vi "DQMH_API_Get All Events in Module.vi"(7 "include all events (F)":bool, 8 "error in (no error)":errorcluster, 11 "Module Info":T1) -> (0 "error out":errorcluster, 3 "Event Info":T2(array[cluster]))   [LabVIEW 2020]
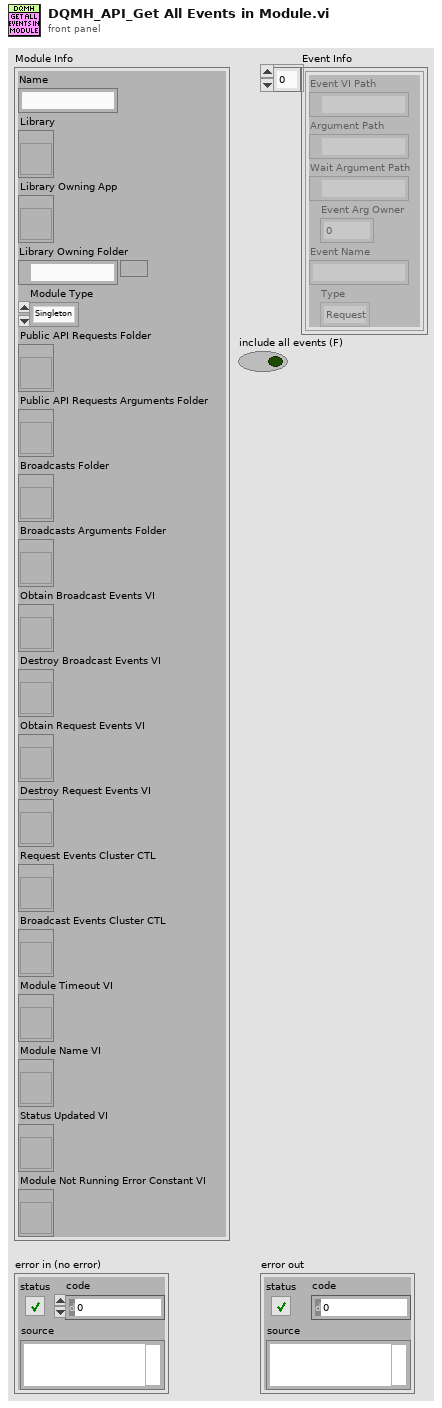
[diagram p1: front panel]
types:
  T1 = cluster{"Name":string, "Library":refnum<vi>, "Library Owning App":refnum<vi>, "Library Owning Folder":path, "Module Type":enum16{"Singleton", "Cloneable"}, "Public API Requests Folder":refnum<vi>, "Public API Requests Arguments Folder":refnum<vi>, "Broadcasts Folder":refnum<vi>, "Broadcasts Arguments Folder":refnum<vi>, "Obtain Broadcast Events VI":refnum<vi>, "Destroy Broadcast Events VI":refnum<vi>, "Obtain Request Events VI":refnum<vi>, "Destroy Request Events VI":refnum<vi>, "Request Events Cluster CTL":refnum<vi>, "Broadcast Events Cluster CTL":refnum<vi>, "Module Timeout VI":refnum<vi>, "Module Name VI":refnum<vi>, "Status Updated VI":refnum<vi>, "Module Not Running Error Constant VI":refnum<vi>}
  T2 = cluster{"Event VI Path":path, "Argument Path":path, "Wait Argument Path":path, "Event Arg Owner":i32, "Event Name":string, "Type":enum16{"Request", "Broadcast", "Both"}}[]
  T3 = typedef "DQMH New Unit Test.lvlib/Event Info.ctl" = cluster{"Event VI Path":path, "Argument Path":path, "Wait Argument Path":path, "Event Arg Owner":i32, "Event Name":string, "Type":T4}
  T4 = typedef "DQMH New Unit Test.lvlib/Event Type.ctl" = enum16{"Request", "Broadcast", "Both"}
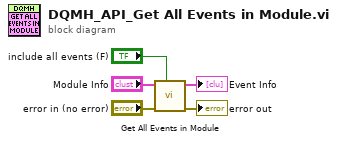
[diagram p0: block diagram]
diagram:
  n1 = call "Get All Events in Module.vi"("include all events (F)"="include all events (F)", "error in (no error)"="error in (no error)", "DQMH Module"="Module Info") -> ("error out"=→"error out":errorcluster, "Event Info"=→"Event Info":T3[])  [unwired: 6 in, 1 out]
